vi "HWPing.vi"(6 "Legacy (f)?":bool, 8 "error in (no error)":errorcluster) -> (0 "error out":errorcluster)   [LabVIEW 2011]
doc: "Ping the hardware engine to make sure the connection is still alive. This VI will error if the connection has been destroyed."
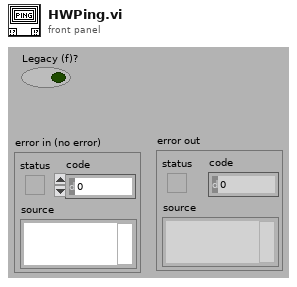
[diagram p1: front panel]
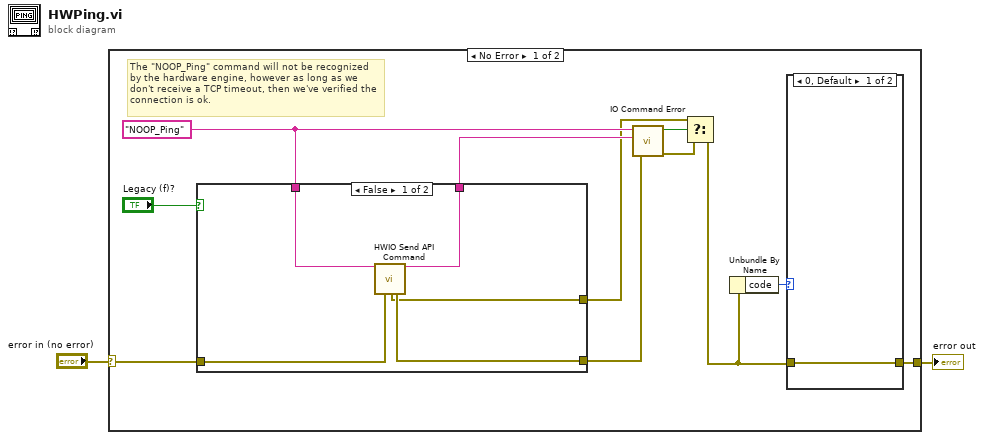
[diagram p0: block diagram]
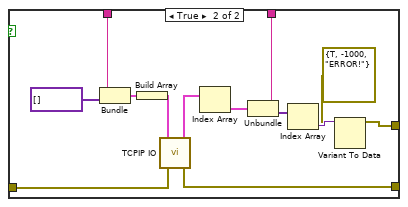
[diagram p2: hidden frame]
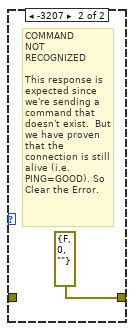
[diagram p3: hidden frame]
diagram:
  n1 = case shown="No Error" "error in (no error)" {
    selector: "error in (no error)" -> [w3 w34]
    tunnel: [w8 w34] -> w2
    frame No Error {
      w12 = "NOOP_Ping"
      # "The \"NOOP_Ping\" command will not be recognized by the hardware engine, however as long as we don't receive a TCP timeout, then we've verified the connection is ok."
      n2 = case shown="False" "Legacy (f)?" {
        tunnel: w3 -> [w18 w31]
        tunnel: [w17 w29] -> w13
        tunnel: w12 -> [w15 w28]
        tunnel: [w16 w25] -> w11
        tunnel: [w14 w19] -> w6
        frame False {
          n3 = call "HWIO Send API Command.vi"("Action"=w15, "error in (no error)"=w18) -> ("Action out"=w16:string, "HWError"=w14:errorcluster, "error out"=w17:errorcluster)  [unwired: 6 in, 5 out]
        }
        frame True {
          n4 = Bundle(w28, "appended array"=variant[] []) -> (w30:cluster{string, "appended array":variant[]})  [unwired: 1 out]
          n5 = Build Array(w30) -> (w27:cluster{string, "appended array":variant[]}[])
          n6 = call "TCPIP IO.vi"("error in (no error)"=w31, "Commands"=w27) -> ("error out"=w29:errorcluster, "Responses"=w24:cluster{string, variant[]}[])  [unwired: 1 in, 3 out]
          n7 = Index Array(array=w24) -> (element=w26:cluster{string, variant[]})  [unwired: 1 in]
          n8 = Unbundle(w26) -> (w25:string, w21:variant[])
          n9 = Index Array(array=w21) -> (element=w23:variant)  [unwired: 1 in]
          n10 = Variant To Data(type=errorcluster {"status"=TRUE, "code"=-1000, "source"="ERROR!"} ("error out"), Variant=w23) -> (data=w19:errorcluster)  [unwired: 1 in, 1 out]
        }
      }
      n11 = call "IO Command Error.vi"("error in (no error)"=w13, "Command Returned (\"\")"=w11, "Command Sent (\"\")"=w12) -> ("error out"=w10:errorcluster, "HW ERR?"=w5:bool)  [unwired: 3 out]
      n12 = Select(t=w6, s=w5, f=w10) -> (s? t:f=w7:errorcluster)
      n13 = Unbundle By Name(w7) -> ("code"=w9:i32)
      n14 = case shown="0, Default" w9 {
        tunnel: w7 -> [w32 _]
        tunnel: [w32 errorcluster {"status"=FALSE, "code"=0, "source"=""} ("error out")] -> w8
        frame 0, Default {
        }
        frame -3207 {
          # "COMMAND\nNOT\nRECOGNIZED\n\nThis response is expected since we're sending a command that doesn't exist.  But we have proven that the connection is still alive (i.e. PING=GOOD). So Clear the Error."
        }
      }
    }
    frame Error {
    }
  }
  "error out" <- w2
